vi "Save Network to File.vi"(0 "Neural Network In":refnum<class "Neural Network.lvclass">, 5 "File Path (dialog)":path, 11 "Error In":errorcluster) -> (6 "Path Used":path, 10 "Cancelled":bool, 15 "Error Out":errorcluster)   [LabVIEW 2015, in "Neural Network.lvclass"]
doc: "Save the neural network to a user editable INI file."
uses:
  Neural Network.lvclass
  <vilib>/Utility/config.llb/NI_LVConfig.lvlib
  <vilib>/Utility/config.llb/Write Key (U32).vi
  <vilib>/Utility/config.llb/Write Key (String).vi
  <vilib>/Utility/config.llb/Write Key (Boolean).vi
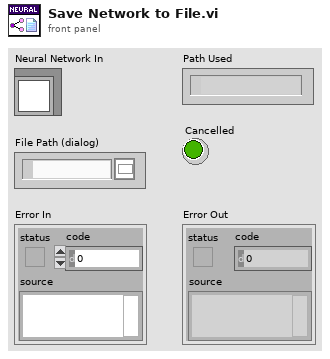
[diagram p1: front panel]
types:
  T1 = enum16{"open", "replace", "create", "open or create", "replace or create", "replace or create with confirmation"}
  T2 = typedef "NI_LVConfig.lvlib/Config Data RefNum.ctl" = refnum<k1>
  T3 = typedef "Neural Network.lvclass/2D Array.ctl" = cluster{"2D Array":sgl[][]}
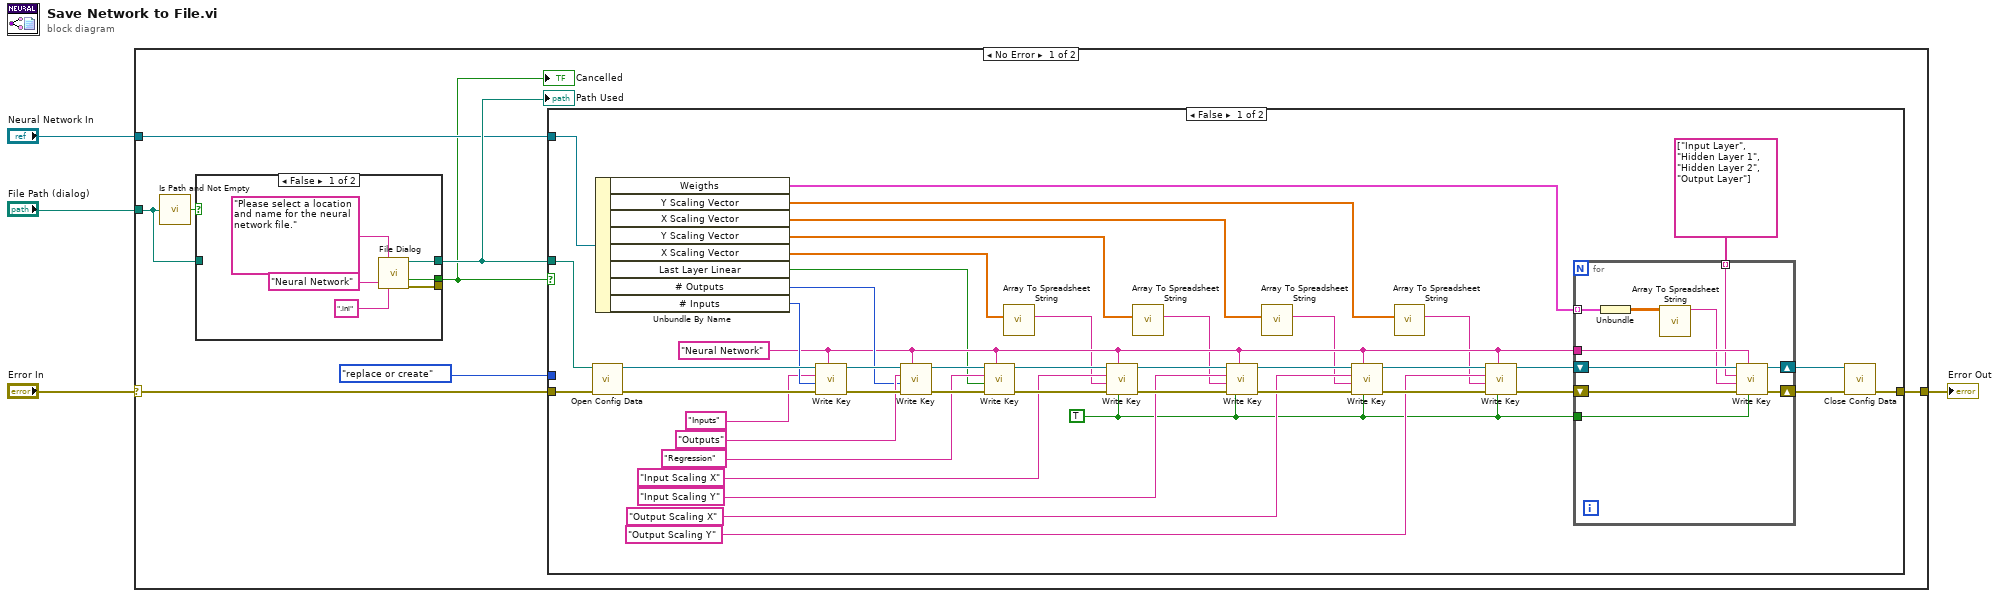
[diagram p0: block diagram]
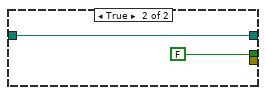
[diagram p3: hidden frame]
diagram:
  n1 = case shown="No Error" "Error In" {
    selector: "Error In" -> [w10 w76]
    tunnel: [w8 w76] -> w3
    tunnel: "Neural Network In" -> [w9 _]
    tunnel: "File Path (dialog)" -> [w7 _]
    frame No Error {
      n2 = call <vilib>:"Is Path and Not Empty.vi"("path"=w7) -> ("Is Path and Not Empty?"=w12:bool)  [unwired: 4 in]
      n3 = case shown="False" w12 {
        tunnel: [w70 w75] -> w11
        tunnel: w7 -> [_ w75]
        tunnel: [w69 FALSE ("cancelled")] -> w6
        tunnel: [w68 _] -> _
        frame False {
          n4 = call "File Dialog"("prompt"="Please select a location and name for the neural network file.", "pattern (all files)"=".ini", "pattern label"="Neural Network") -> ("selected path"=w70:path, "cancelled"=w69:bool, "error out"=w68:errorcluster)  [unwired: 9 in, 1 out]
        }
        frame True {
        }
      }
      "Cancelled" <- w6
      "Path Used" <- w11
      n5 = case shown="False" w6 {
        tunnel: w11 -> [w55 _]
        tunnel: w10 -> [w56 w67]
        tunnel: w9 -> [w23 _]
        tunnel: [w37 w67] -> w8
        tunnel: T1."replace or create" ("operation (0:open)") -> [_ _]
        frame False {
          w21 = TRUE ("write raw string? (F)")
          w25 = "Neural Network" ("section")
          n6 = call <vilib>:"Open Config Data.vi"("error in (no error)"=w56, "configuration file path"=w55) -> ("error out"=w53:errorcluster, "refnum"=w54:T2)  [unwired: 7 in, 1 out]
          n7 = Unbundle By Name(w23) -> ("Weigths"=w26:T3[], "Y Scaling Vector"=w14:dbl[], "X Scaling Vector"=w16:dbl[], "Y Scaling Vector"=w18:dbl[], "X Scaling Vector"=w20:dbl[], "Last Layer Linear"=w22:bool, "# Outputs"=w47:u32, "# Inputs"=w52:u32)
          n8 = call-poly <vilib>:"Write Key.vi"("section"=w25, "error in (no error)"=w53, "value"=w52, "key"="Inputs", "refnum"=w54) -> ("error out"=w50:errorcluster, "refnum out"=w51:T2)  [unwired: 4 in, 1 out]
          n9 = call-poly <vilib>:"Write Key.vi"("section"=w25, "error in (no error)"=w50, "value"=w47, "key"="Outputs", "refnum"=w51) -> ("error out"=w45:errorcluster, "refnum out"=w46:T2)  [unwired: 4 in, 1 out]
          n10 = call-poly <vilib>:"Write Key.vi"("section"=w25, "error in (no error)"=w45, "value"=w22, "key"="Regression", "refnum"=w46) -> ("error out"=w44:errorcluster, "refnum out"=w41:T2)  [unwired: 4 in, 1 out]
          n11 = call "Array To Spreadsheet String.vi"("1D Array"=w20) -> ("1D Spreadsheet String"=w19:string)  [unwired: 9 in, 1 out]
          n12 = call-poly <vilib>:"Write Key.vi"("write raw string? (F)"=w21, "section"=w25, "error in (no error)"=w44, "value"=w19, "key"="Input Scaling X", "refnum"=w41) -> ("error out"=w42:errorcluster, "refnum out"=w38:T2)  [unwired: 3 in, 1 out]
          n13 = call "Array To Spreadsheet String.vi"("1D Array"=w18) -> ("1D Spreadsheet String"=w17:string)  [unwired: 9 in, 1 out]
          n14 = call-poly <vilib>:"Write Key.vi"("write raw string? (F)"=w21, "section"=w25, "error in (no error)"=w42, "value"=w17, "key"="Input Scaling Y", "refnum"=w38) -> ("error out"=w39:errorcluster, "refnum out"=w34:T2)  [unwired: 3 in, 1 out]
          n15 = call "Array To Spreadsheet String.vi"("1D Array"=w16) -> ("1D Spreadsheet String"=w15:string)  [unwired: 9 in, 1 out]
          n16 = call-poly <vilib>:"Write Key.vi"("write raw string? (F)"=w21, "section"=w25, "error in (no error)"=w39, "value"=w15, "key"="Output Scaling X", "refnum"=w34) -> ("error out"=w35:errorcluster, "refnum out"=w31:T2)  [unwired: 3 in, 1 out]
          n17 = call "Array To Spreadsheet String.vi"("1D Array"=w14) -> ("1D Spreadsheet String"=w13:string)  [unwired: 9 in, 1 out]
          n18 = call-poly <vilib>:"Write Key.vi"("write raw string? (F)"=w21, "section"=w25, "error in (no error)"=w35, "value"=w13, "key"="Output Scaling Y", "refnum"=w31) -> ("error out"=w32:errorcluster, "refnum out"=w28:T2)  [unwired: 3 in, 1 out]
          n19 = for {
            shift-right: [w65] -> w29
            shift-left: w32 -> [w66]
            shift-right: [w63] -> w27
            shift-left: w28 -> [w64]
            tunnel: w26 -> [w62] mode=indexing
            tunnel: w25 -> [w61]
            tunnel: string[] ["Input Layer", "Hidden Layer 1", "Hidden Layer 2", "Output Layer"] -> [w60] mode=indexing
            tunnel: w21 -> [w59]
            n20 = Unbundle(w62) -> ("2D Array"=w58:sgl[][])
            n21 = call "Array To Spreadsheet String.vi"("2D Array"=w58) -> ("2D Spreadsheet String"=w57:string)  [unwired: 9 in, 1 out]
            n22 = call-poly <vilib>:"Write Key.vi"("write raw string? (F)"=w59, "section"=w61, "error in (no error)"=w66, "value"=w57, "key"=w60, "refnum"=w64) -> ("error out"=w65:errorcluster, "refnum out"=w63:T2)  [unwired: 3 in, 1 out]
          }
          n23 = call <vilib>:"Close Config Data.vi"("error in (no error)"=w29, "refnum"=w27) -> ("error out"=w37:errorcluster)  [unwired: 8 in, 1 out]
        }
        frame True {
        }
      }
    }
    frame Error {
    }
  }
  "Error Out" <- w3
